vi "auto.vi"() -> ()   [LabVIEW 2017]
panel:
  in  "User Name":string
  in  "LOGIN":string
  out "LOGIN SUSSESS":bool
  in  "A2_HMI_SEND_ 3":i32
  in  "A2_HMI_SEND_ 2":i32
  in  "A2_HMI_SEND_1":i32
  in  "A1_HMI_SEND_ 3":i32
  in  "A1_HMI_SEND_ 2":i32
  in  "A1_HMI_SEND_1":i32
  out "SCANNER 13":string
  out "SCANNER 12":string
  out "SCANNER 11":string
  out "SCANNER 10":string
  out "SCANNER 9":string
  out "SCANNER 8":string
  out "SCANNER 7":string
  out "SCANNER 6":string
  out "SCANNER 5":string
  out "SCANNER 4":string
  out "SCANNER 3":string
  out "SCANNER 2":string
  out "SCANNER 1":string
  out "ASSEMBLY 1_01":T1
  # "Assembly 1-01"
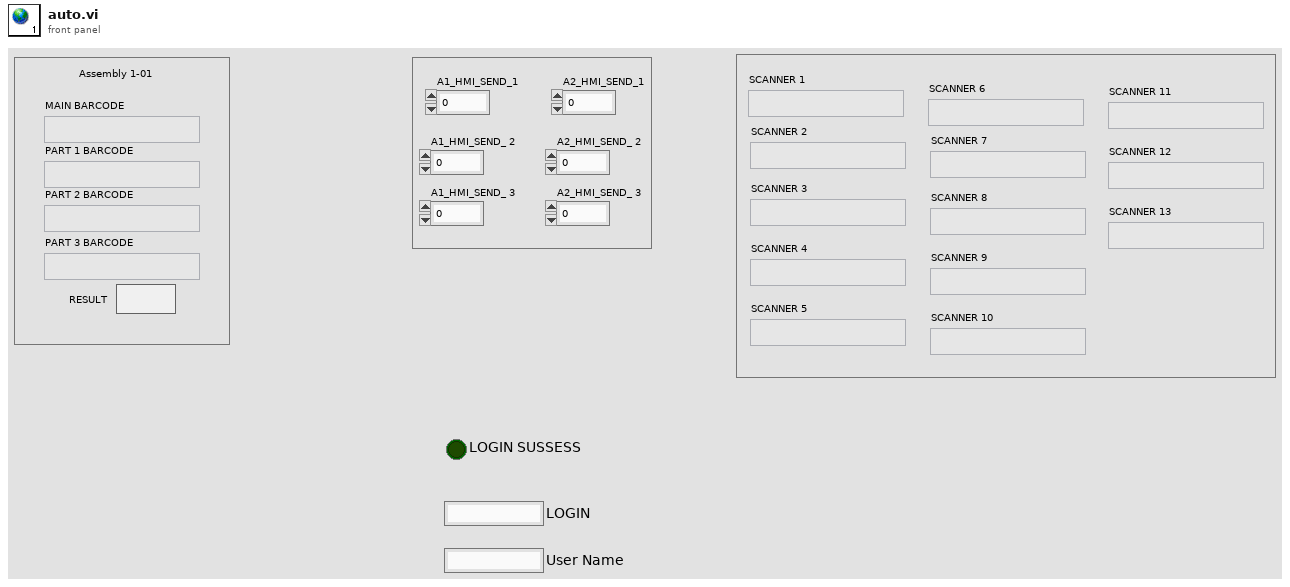
[diagram p1: front panel]
types:
  T1 = cluster{"MAIN BARCODE":string, "PART 1 BARCODE":string, "PART 2 BARCODE":string, "PART 3 BARCODE":string, "RESULT":bool}
diagram:
